vi "Choose View Type.vi"(8 "error in (no error)":errorcluster, 11 "Example Controller Actor in":refnum<class "Example Controller Actor.lvclass">) -> (0 "error out":errorcluster, 3 "Example Controller Actor out":refnum<class "Example Controller Actor.lvclass">)   [LabVIEW 2023, in "Example GUI View Actor.lvlib" / "Example Controller Actor.lvclass"]
uses:
  Example Controller Actor.lvclass
  Example GUI View Actor/Example GUI View Actor.lvclass
  Example Controller Actor.lvclass/Example Controller Actor.ctl
  GUI Views/GUI View Actor/GUI View Actor.lvclass/GUI View Actor.ctl
  Example Controller Actor/Example Controller Actor/Example Controller Actor.lvclass/Example Controller Actor.ctl
  GUI Views/GUI View Actor/properties/Write Container Enqueuer.vi
  Example Controller Actor/Example Controller Actor/properties/Write View Type.vi
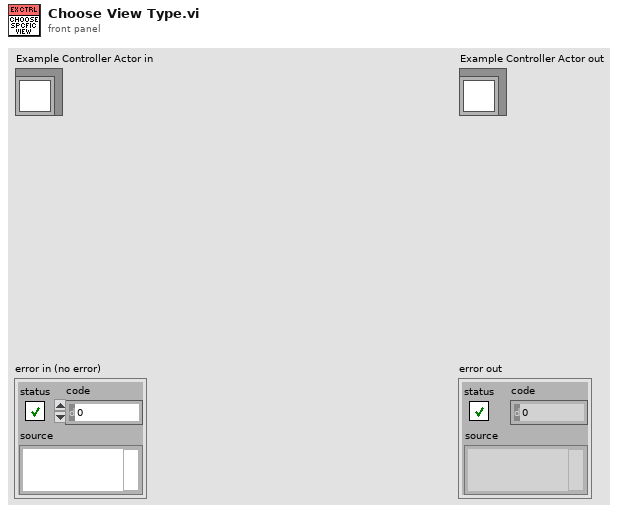
[diagram p1: front panel]
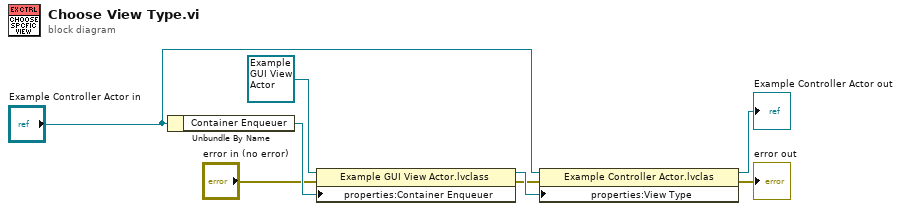
[diagram p0: block diagram]
diagram:
  n1 = Unbundle By Name("Example Controller Actor in") -> ("Container Enqueuer"=w3:refnum<class "Message Enqueuer.lvclass">)
  n2 = property class="Example GUI View Actor.lvclass"(reference=refnum<class "Example GUI View Actor.lvclass"> refnum ("Example GUI View Actor.lvlib:Example GUI View Actor.lvclass"), error in="error in (no error)", "properties:Container Enqueuer"=w3) -> (reference out=w5:refnum<class "Example GUI View Actor.lvclass">, error out=w1:errorcluster)
  n3 = property class="Example Controller Actor.lvclas"(reference="Example Controller Actor in", error in=w1, "properties:View Type"=w5) -> (reference out=→"Example Controller Actor out":refnum<class "Example Controller Actor.lvclass">, error out=→"error out":errorcluster)
